vi "Exercice 5.vi"() -> ()   [LabVIEW 2018]
panel:
  in  "Débit":i32 min=0 max=10
  in  "?":bool
  in  "Consigne":i32 min=0 max=1000
  out "Tank":i32(slide) scale=0.0..1000.0
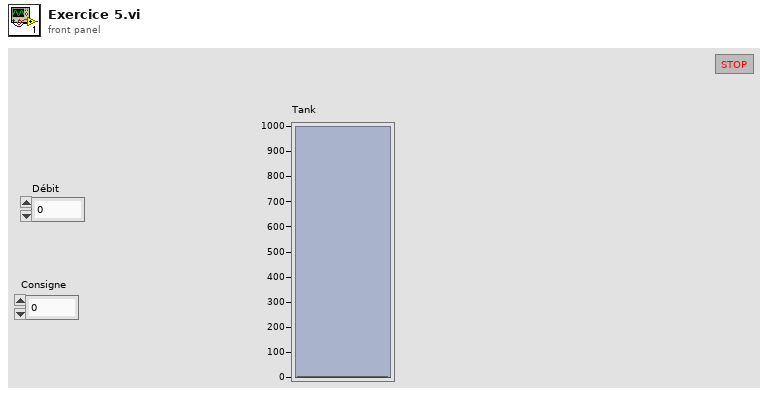
[diagram p1: front panel]
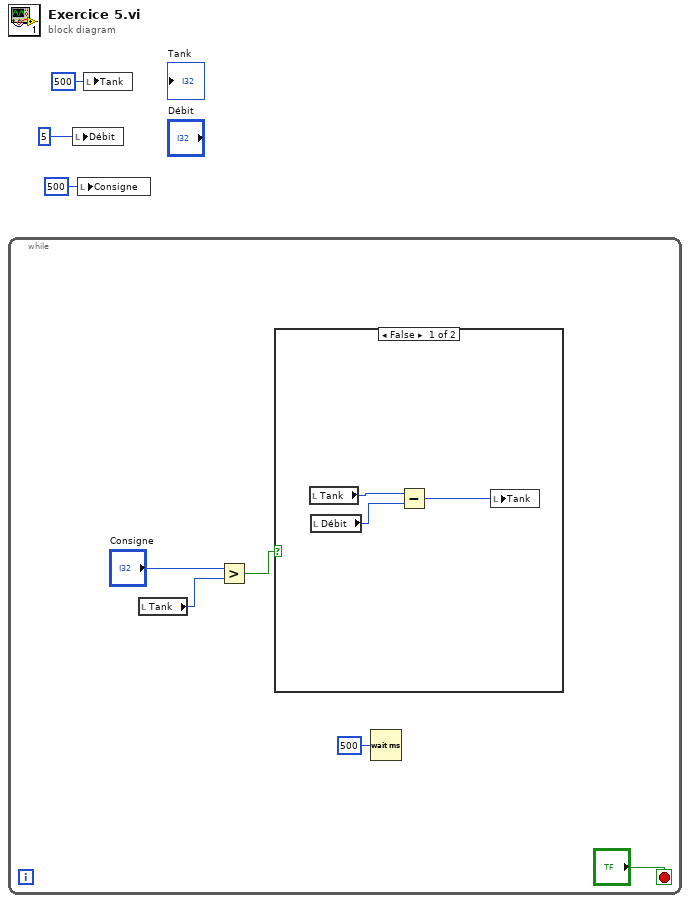
[diagram p0: block diagram]
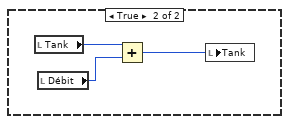
[diagram p2: hidden frame]
diagram:
  n1 = while {
    stop <- "?" stop-if-true
    n2 = local read "Tank"() -> (w6:i32)
    n3 = Greater?(x="Consigne", y=w6) -> (0:w5:bool)
    n4 = case shown="False" w5 {
      frame False {
        n5 = local read "Tank"() -> (w11:i32)
        n6 = local read "Débit"() -> (w9:i32)
        n7 = Subtract(x=w11, y=w9) -> (x-y=w10:i32)
        n8 = local write "Tank"(w10) -> ()
      }
      frame True {
        n9 = local read "Tank"() -> (w13:i32)
        n10 = local read "Débit"() -> (w12:i32)
        n11 = Add(x=w13, y=w12) -> (x+y=w14:i32)
        n12 = local write "Tank"(w14) -> ()
      }
    }
    n13 = Wait (ms)(milliseconds to wait=u32 500) -> ()  [unwired: 1 out]
  }
  n14 = local write "Débit"(5 ("Débit")) -> ()
  n15 = local write "Consigne"(500 ("Consigne")) -> ()
  n16 = local write "Tank"(500 ("Tank")) -> ()
